vi "main.vi"() -> ()   [LabVIEW 2016, in "LabVIEWCodeCoverage.lvlib"]
uses:
  LabVIEWCodeCoverage.lvlib
panel:
  in  "Reset":bool
  in  "Refresh%":bool
  in  "SourcePath":path
  in  "Stop":bool
  in  "Start":bool
  in  "RefreshContext":bool
  in  "Context":u16(ring) items=["<Empty>", "Main Application Instance", "NI.LV.Merge", "src.lvproj My Computer", "src.lvproj My Computer"]
  in  "VITree":string(tree)
  in  "UnCoveredDiagram":i32(listbox)
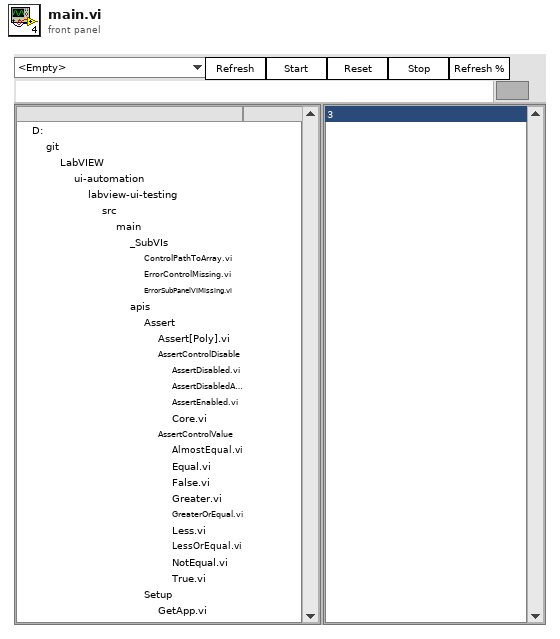
[diagram p1: front panel]
types:
  T1 = enum32{"Invalid", "Standard", "Closed", "Hidden", "Minimized", "Maximized"}
  T2 = enum32{"invalid app kind", "Development System", "Run Time System", "Student Edition", "Embedded LabVIEW", "Evaluation", "Custom"}
  T3 = cluster{"Context":string, "Project":string, "Display":string, "ProjectPath":path}
  T4 = cluster{"Context":string, "Project":string, "Display":string, "ProjectPath":path}[]
  T5 = cluster{"Core":cluster{"Current VI Reference":refnum<vi>, "Close Panel on Exit?":bool}, "ActiveContext":string, "Context[]":cluster{"Context":string, "Project":string, "Display":string, "ProjectPath":path}[], "SourcePath":path, "SourceFiles[]":path[], "ActiveVI":string, "Uncovered Diagrams":refnum<vi>[], "ActiveVIRef":refnum<vi>}
  T6 = cluster{"Current VI Reference":refnum<vi>, "Close Panel on Exit?":bool}
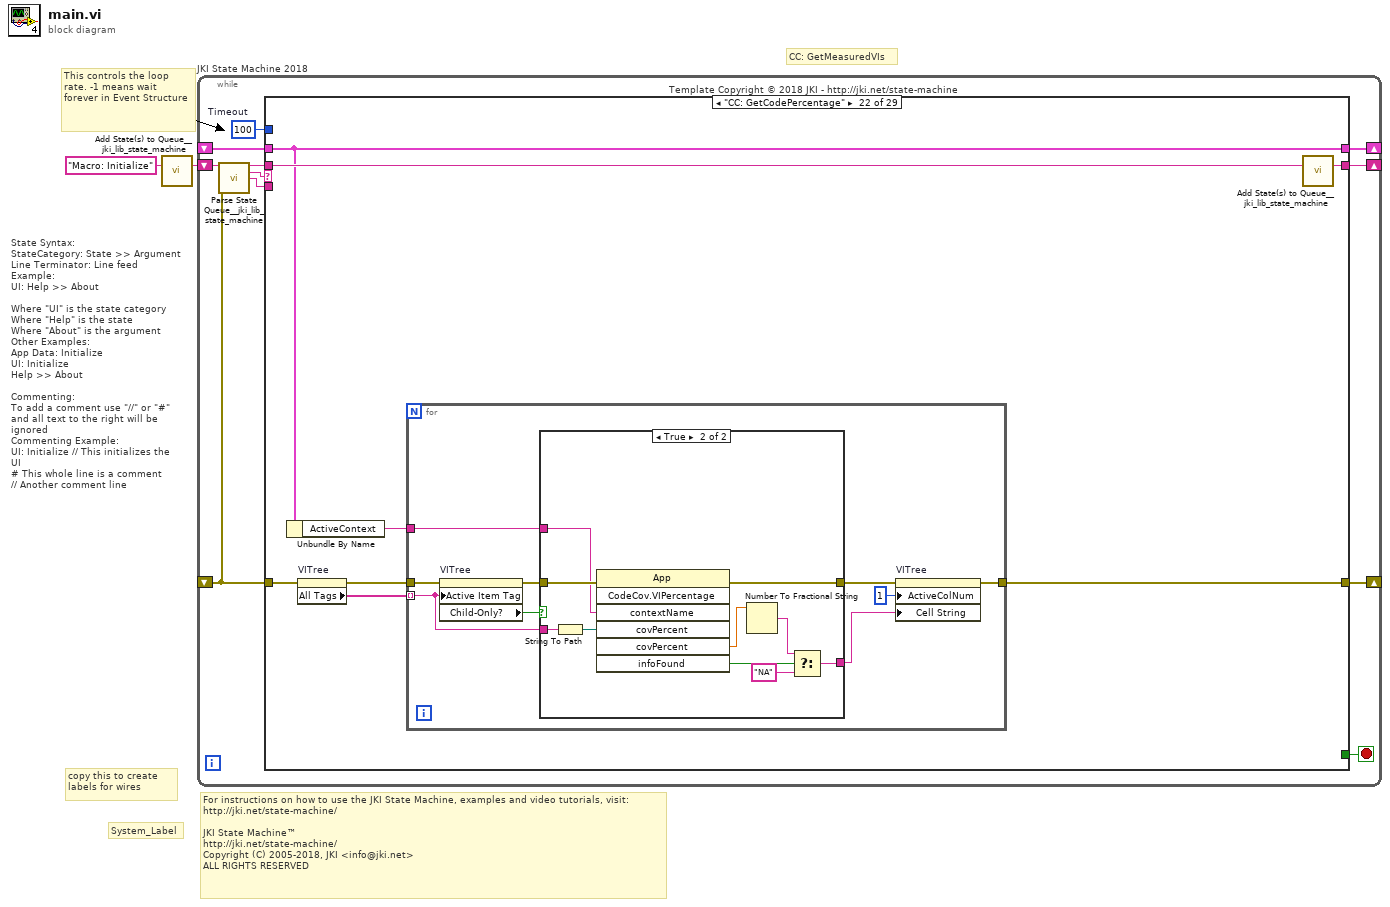
[diagram p0: block diagram]
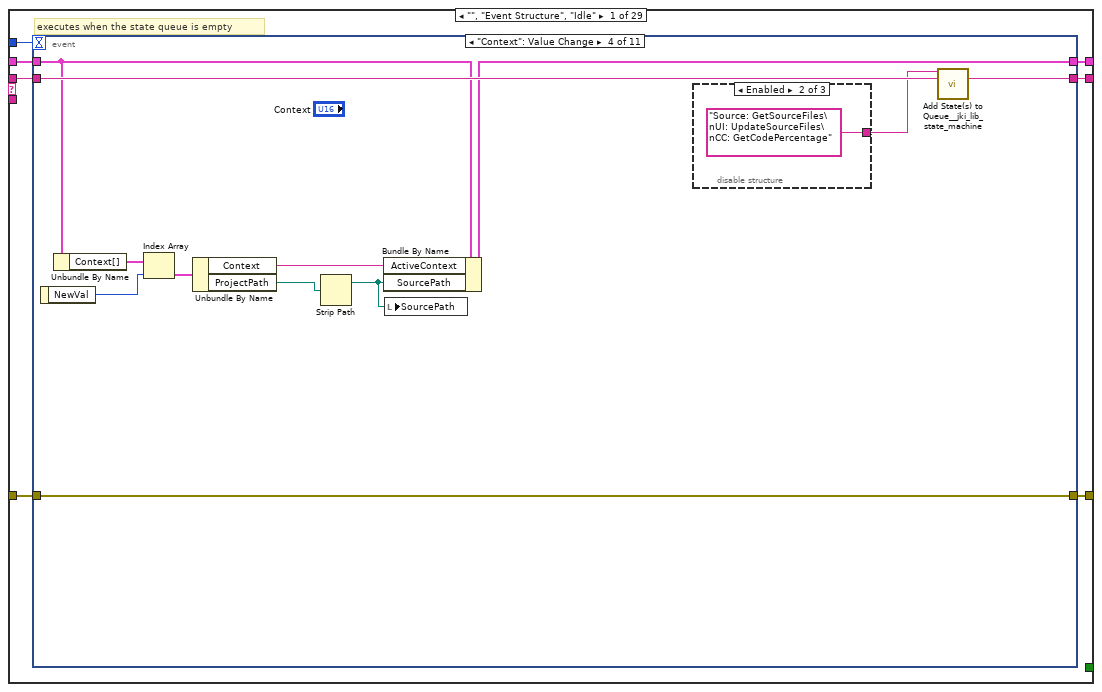
[diagram p2: hidden frame]
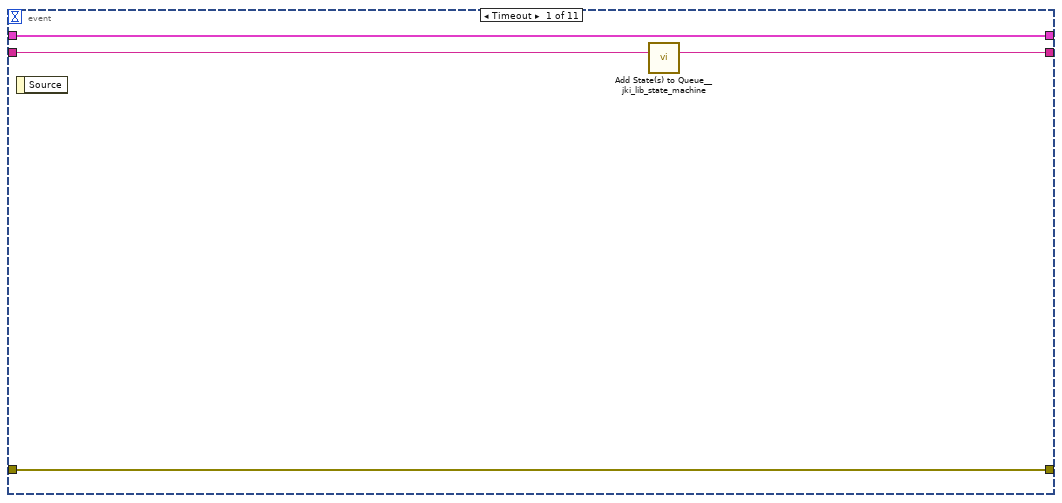
[diagram p3: hidden frame]
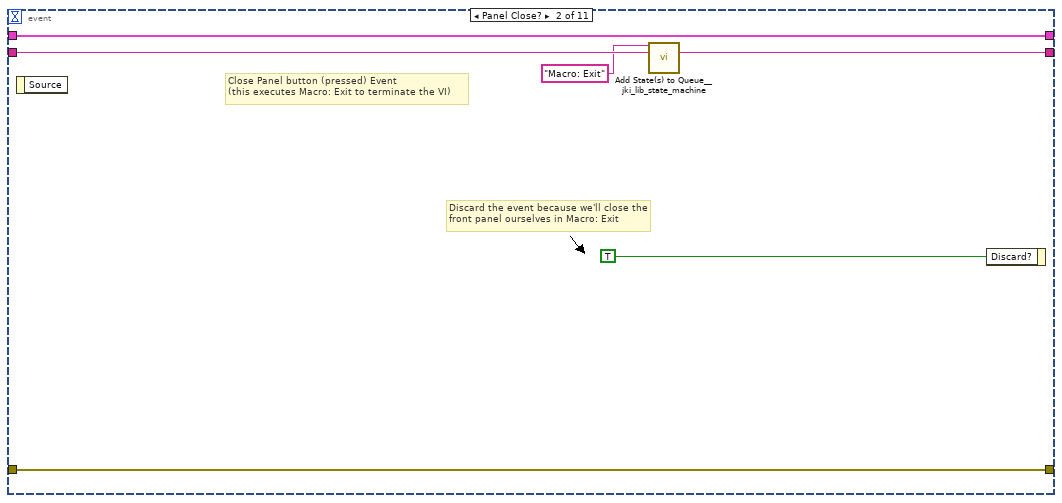
[diagram p4: hidden frame]
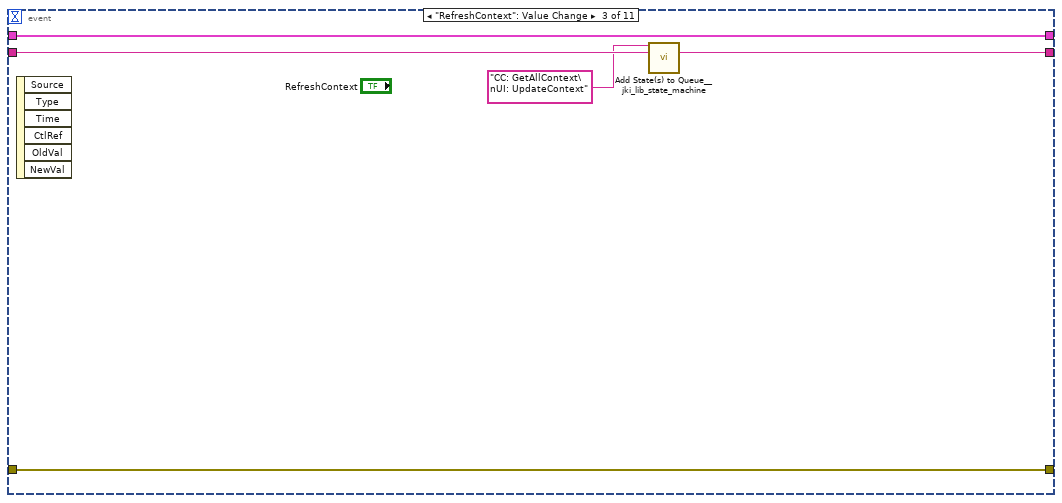
[diagram p5: hidden frame]
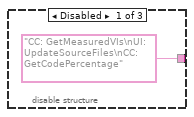
[diagram p6: hidden frame]
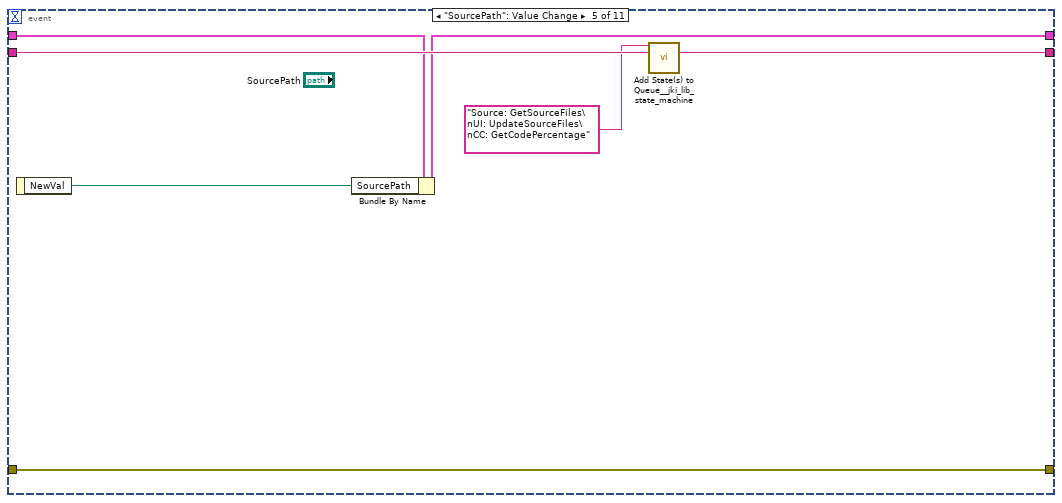
[diagram p8: hidden frame]
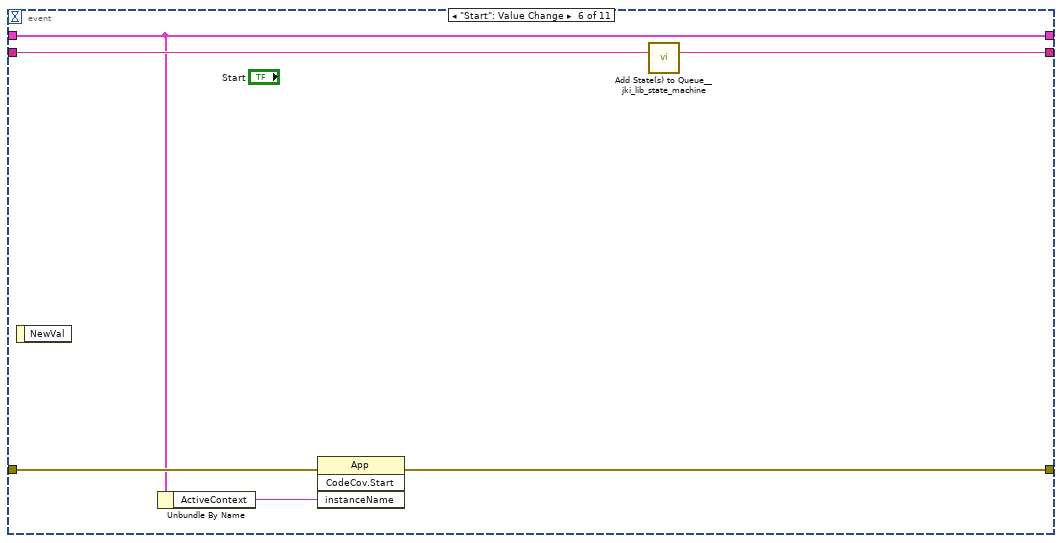
[diagram p9: hidden frame]
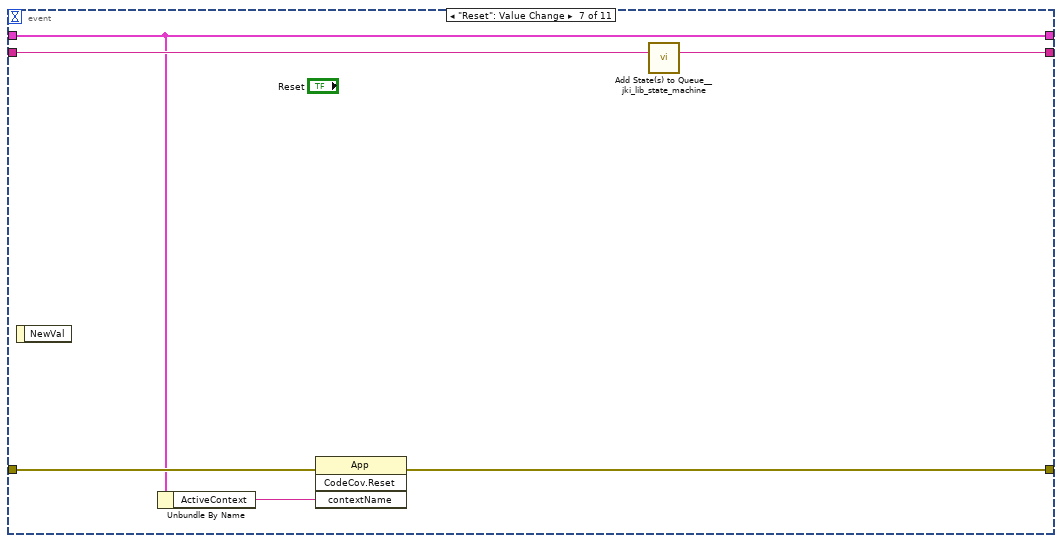
[diagram p10: hidden frame]
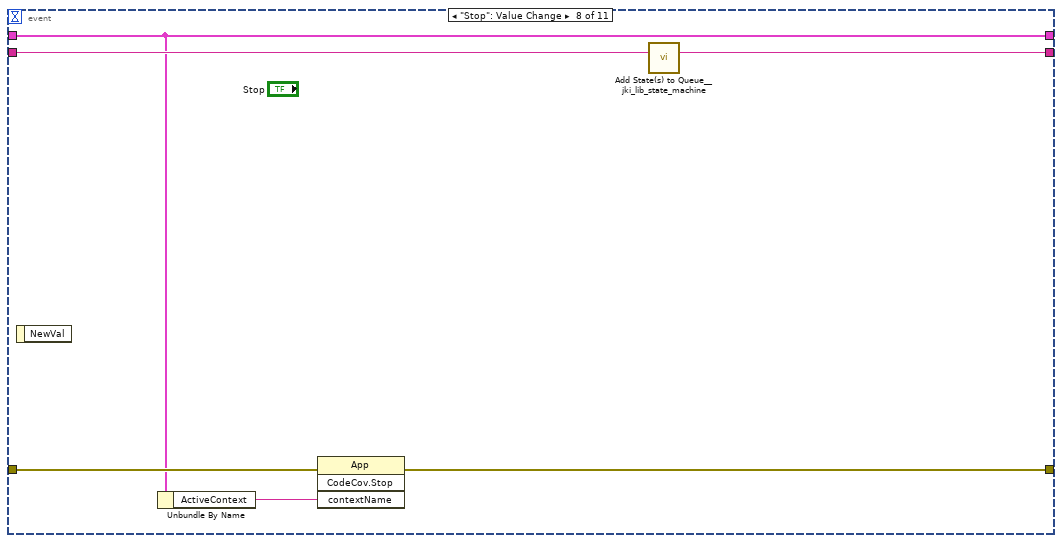
[diagram p11: hidden frame]
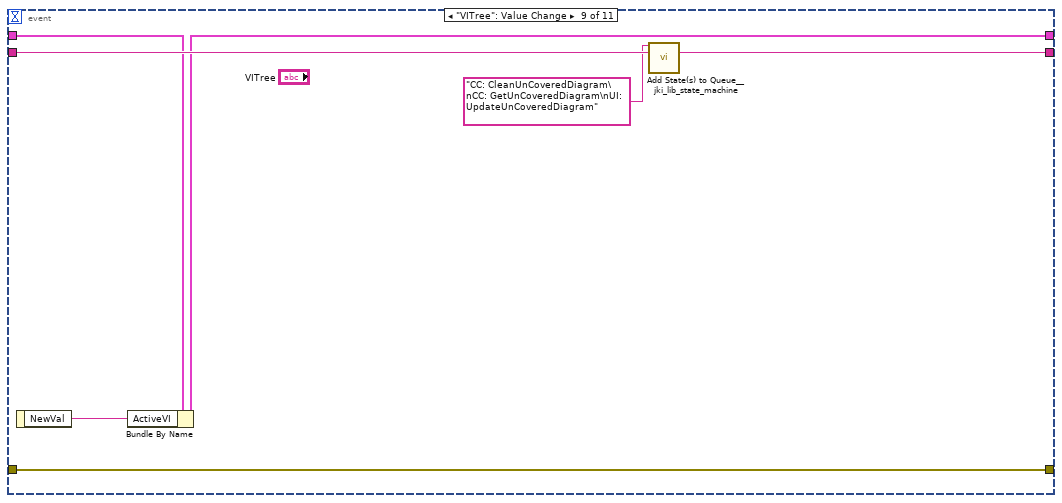
[diagram p12: hidden frame]
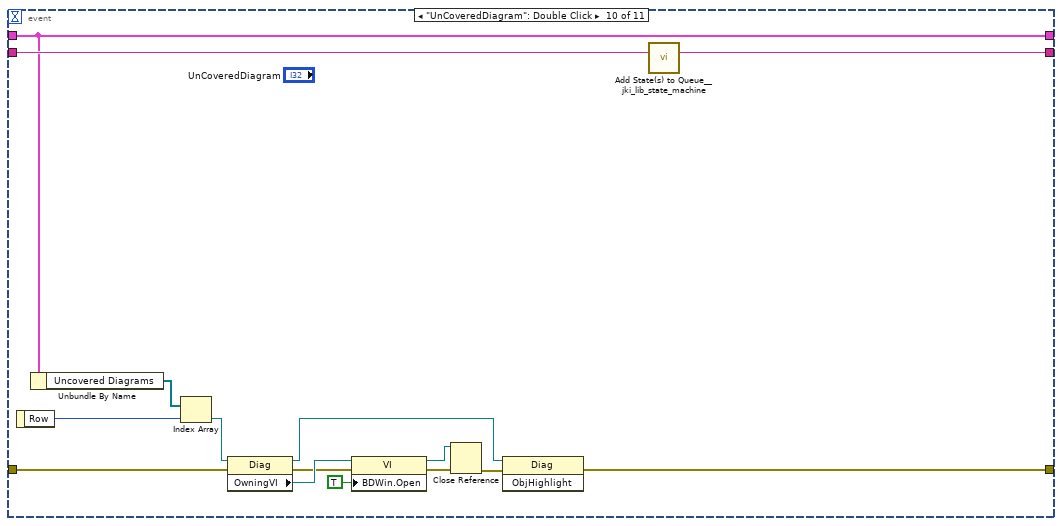
[diagram p13: hidden frame]
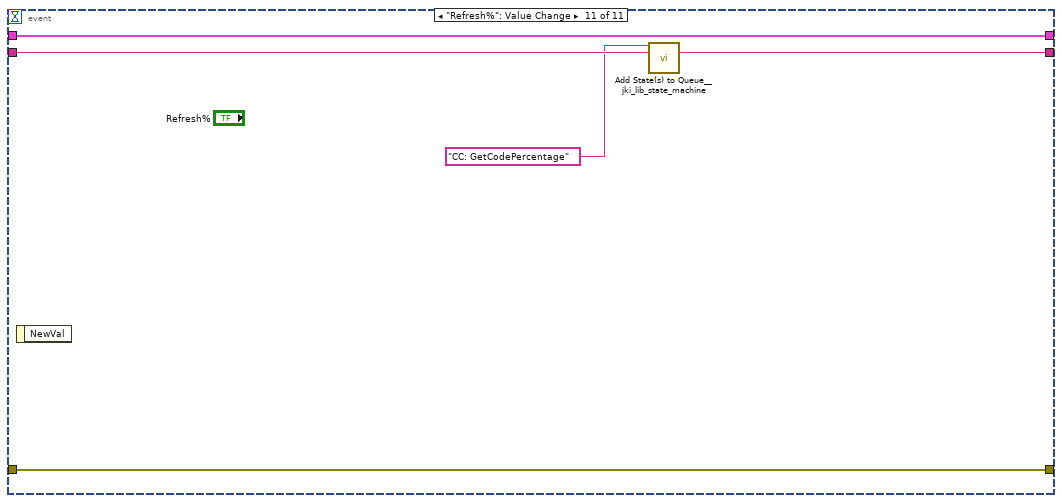
[diagram p14: hidden frame]
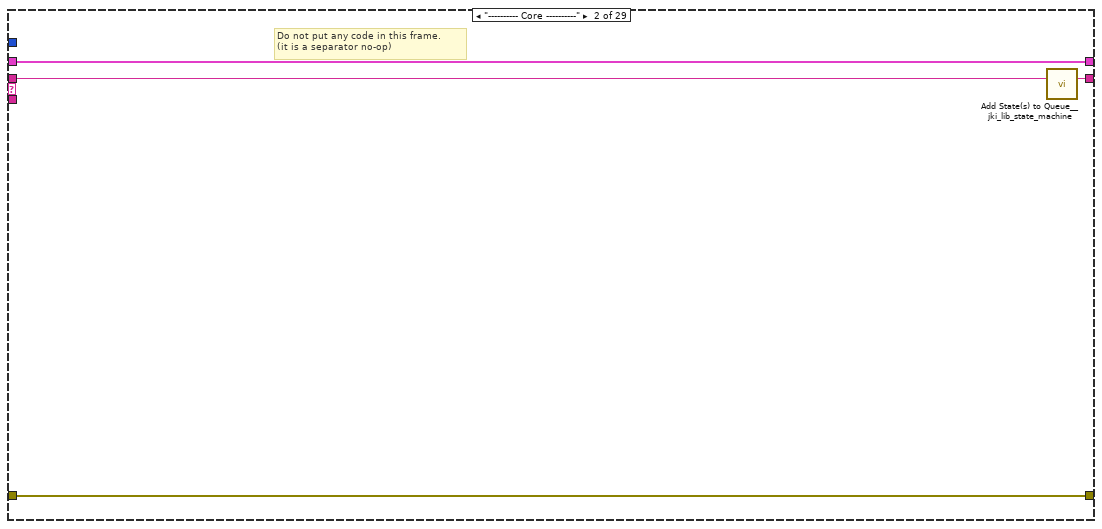
[diagram p15: hidden frame]
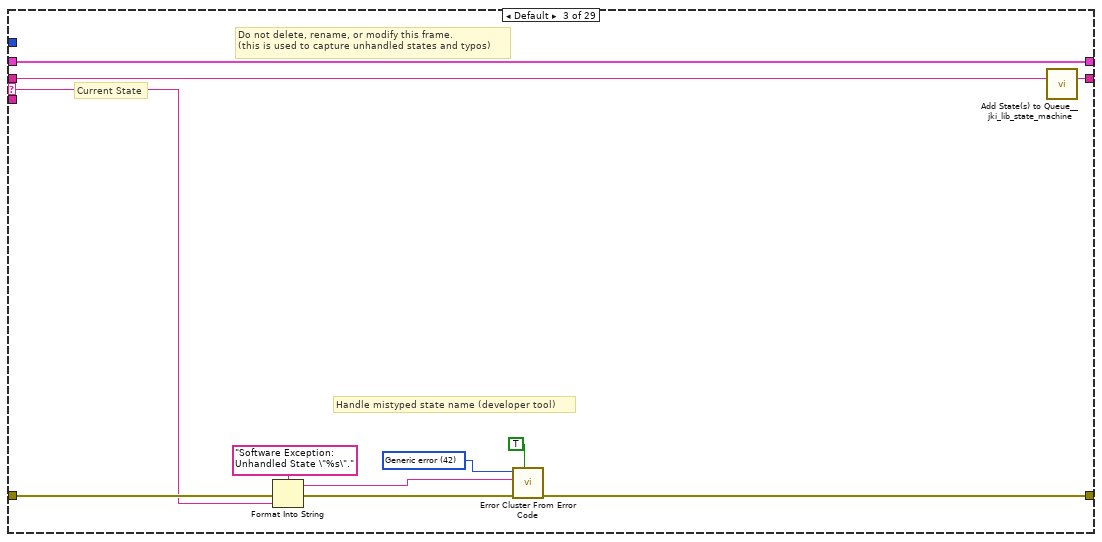
[diagram p16: hidden frame]
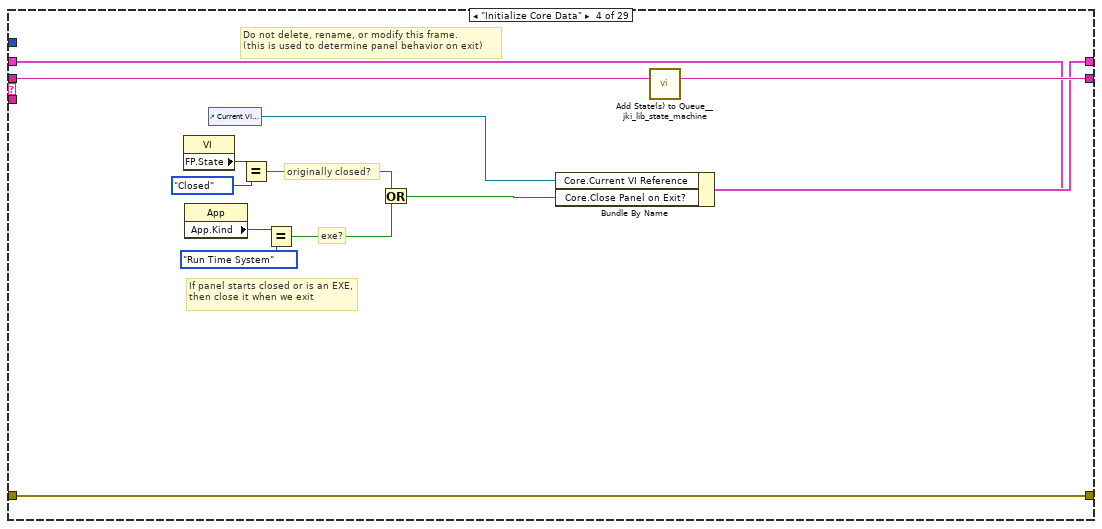
[diagram p17: hidden frame]
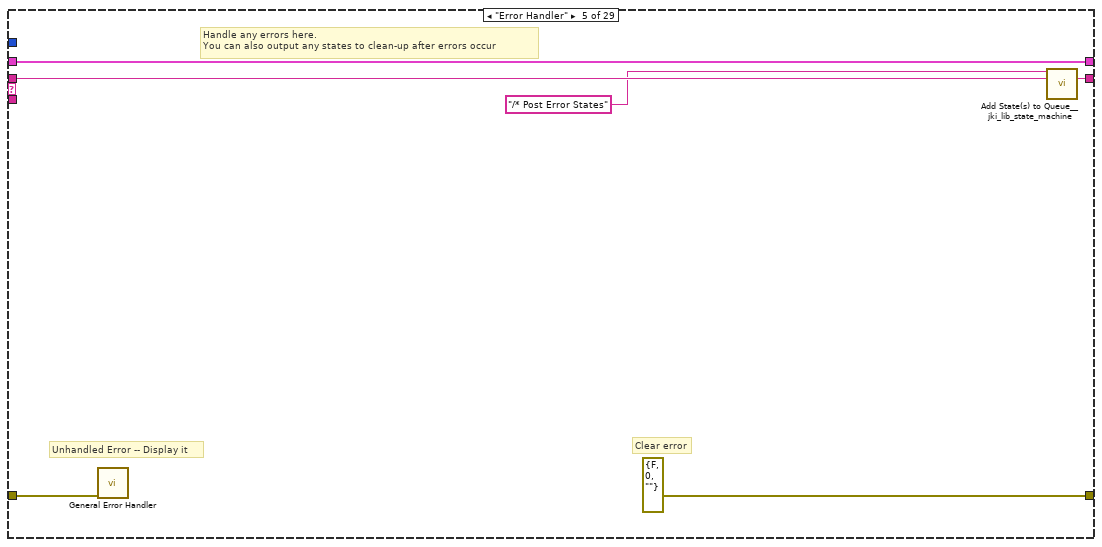
[diagram p18: hidden frame]
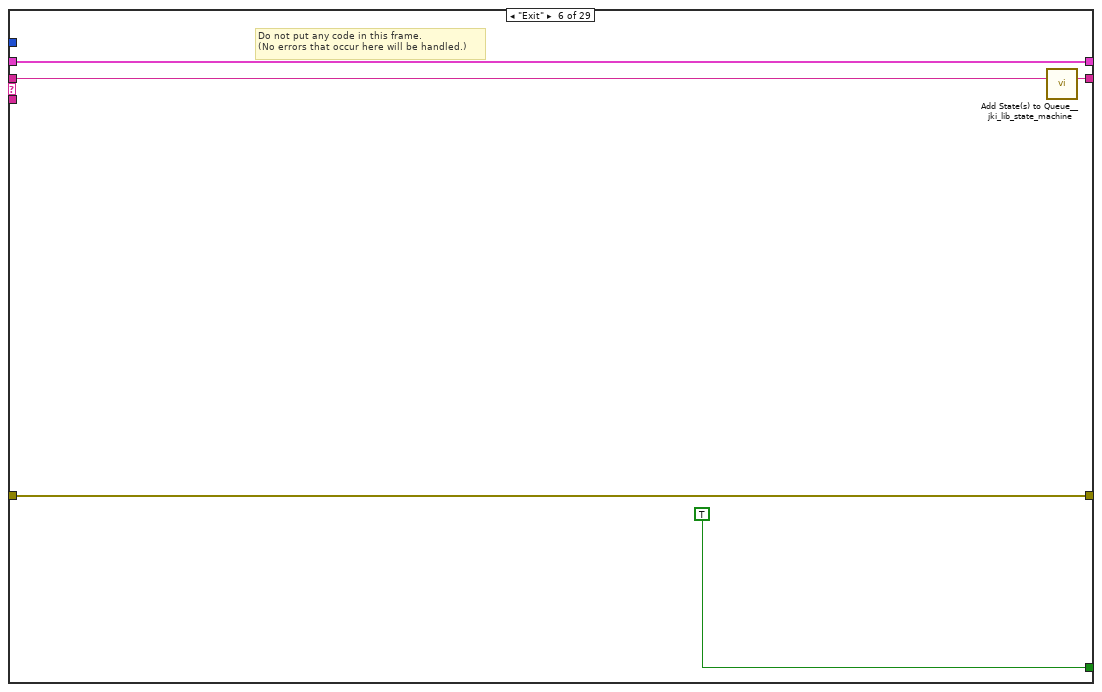
[diagram p19: hidden frame]
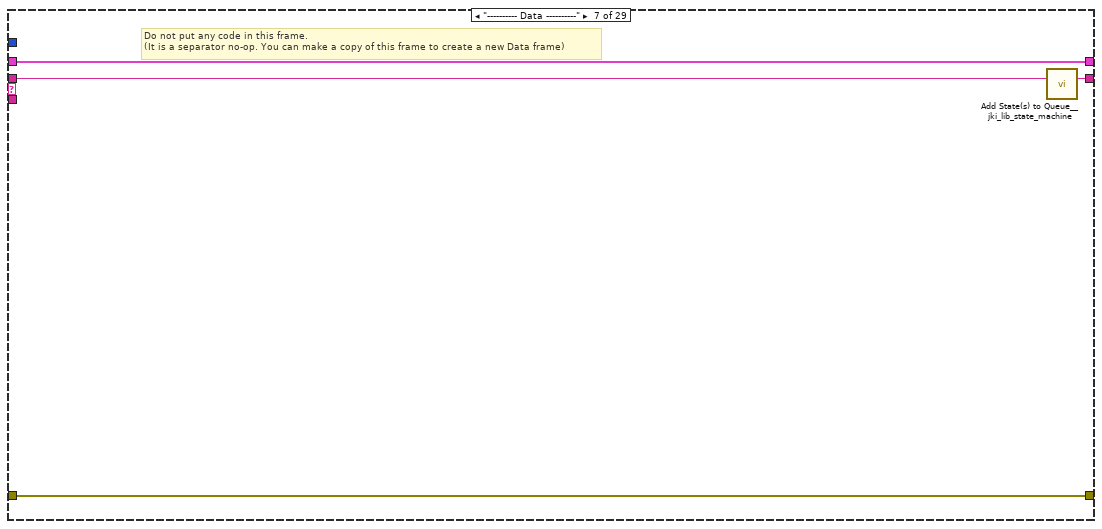
[diagram p20: hidden frame]
diagram:
  # "CC: GetMeasuredVIs"
  # "For instructions on how to use the JKI State Machine, examples and video tutorials, visit:\nhttp://jki.net/state-machine/\n\nJKI State Machine™\nhttp://jki.net/state-machine/\nCopyright (C) 2005-2018, JKI <info@jki.net>\nALL RIGHTS RESERVED"
  # "State Syntax:\nStateCategory: State >> Argument\nLine Terminator: Line feed\nExample:\nUI: Help >> About\n\nWhere \"UI\" is the state category\nWhere \"Help\" is the state\nWhere \"About\" is the argument\nOther Examples:\nApp Data: Initialize\nUI: Initialize\nHelp >> About\n\nCommenting:\nTo add a comment use \"//\" or \"#\" and all text to the right will be ignored\nCommenting Example:\nUI: Initialize // This initializes the UI\n# This whole line is a comment\n// Another comment line"
  # "copy this to create labels for wires"
  # "This controls the loop rate. -1 means wait forever in Event Structure"
  # "System_Label"
  n1 = call <vilib>:"Add State(s) to Queue__jki_lib_state_machine.vi"("State(s) in (\"\")"="Macro: Initialize") -> ("States Out"=w2:string)  [unwired: 14 in]
  n2 = while "JKI State Machine 2018" {
    shift-right: [w6] -> _
    shift-left: _ -> [w5]
    shift-right: [w9] -> _
    shift-left: _ -> [w3]
    shift-right: [w8] -> _
    shift-left: w2 -> [w10]
    stop <- w7 stop-if-true
    w4 = 100  # Timeout
    # "Template Copyright © 2018 JKI - http://jki.net/state-machine"
    n3 = call <vilib>:"Parse State Queue__jki_lib_state_machine.vi"("State Queue"=w10, "Error In (no error)"=w3) -> ("Remaining States"=w12:string, "Current State"=w13:string, "Arguments"=w11:string)  [unwired: 11 in]
    n4 = case shown="\"CC: GetCodePercentage\"" w13 {
      selector: w13 -> [_ _ w106 _ _ _ _ _ _ _ _ _ _ _ _ _ _ _ _ _ _ _ _ _ _ _ _ _ _]
      tunnel: w12 -> [w20 w105 w110 w129 w135 w140 w144 w156 w162 w166 w173 w179 w190 w262 w283 w302 w312 w317 w327 w331 w346 w362 w392 w421 w425 w429 w433 w444 w459]
      tunnel: w11 -> [_ _ _ _ _ _ _ _ _ _ _ w174 w184 _ _ _ _ _ _ _ _ _ _ _ _ _ _ _ _]
      tunnel: w5 -> [w18 w102 w108 w122 w132 w138 w141 _ w157 w163 w170 w177 w186 w260 w281 w300 w309 w314 w324 w328 w343 w356 w389 w419 w422 w426 w430 w442 w454]
      tunnel: [w17 w103 w112 w126 errorcluster {"status"=FALSE, "code"=0, "source"=""} ("error out") w137 w142 w153 w158 w164 w171 w175 w187 w258 w267 w299 w310 w315 w325 w329 w340 w360 w388 w410 w423 w427 w431 w436 w455] -> w9
      tunnel: w3 -> [w16 w103 w111 w126 w131 w137 w142 w153 w159 w164 w171 w176 w188 w259 w279 w298 w310 w315 w325 w329 w344 w359 w390 w417 w423 w427 w431 w441 w456]
      tunnel: [w19 w104 w109 w128 w134 w139 w143 w155 w161 w165 w172 w178 w189 w261 w282 w301 w311 w316 w326 w330 w345 w361 w391 w420 w424 w428 w432 w443 w458] -> w8
      tunnel: [_ _ _ _ _ TRUE _ _ _ _ _ _ _ _ _ _ _ _ _ _ _ _ _ _ _ _ _ _ _] -> w7
      tunnel: [w15 w102 w108 w127 w132 w138 w141 w154 w157 w163 w170 w177 w186 w260 w281 w300 w309 w314 w324 w328 w341 w356 w387 w418 w422 w426 w430 w437 w457] -> w6
      tunnel: w4 -> [w14 _ _ _ _ _ _ _ _ _ _ _ _ _ _ _ _ _ _ _ _ _ _ _ _ _ _ _ _]
      frame "", "Event Structure", "Idle" {
        # "executes when the state queue is empty"
        n5 = event shown="[3] \"Context\": Value Change" {
          selector: _ -> [_ _ _ _ _ _ _ _ _ _ _]
          dyn-events: _ -> [_ _ _ _ _ _ _ _ _ _ _]
          timeout: w14 -> [_ _ _ _ _ _ _ _ _ _ _]
          tunnel: w20 -> [w24 w30 w35 w47 w56 w62 w68 w74 w81 w96 w101]
          tunnel: [w23 w29 w34 w46 w55 w61 w67 w73 w80 w95 w100] -> w19
          tunnel: w18 -> [w21 w27 w32 w43 w52 w58 w64 w70 w78 w94 w98]
          tunnel: [w22 w28 w33 w45 w54 w59 w65 w71 w79 w91 w99] -> w17
          tunnel: w16 -> [w22 w28 w33 w45 w54 w60 w66 w72 w79 w90 w99]
          tunnel: [w21 w27 w32 w44 w53 w58 w64 w70 w77 w94 w98] -> w15
          event Timeout {
            n6 = event-data() -> ()  [unwired: 1 in, 1 out]
            n7 = call <vilib>:"Add State(s) to Queue__jki_lib_state_machine.vi"("State(s) in (\"\")"=w24) -> ("States Out"=w23:string)  [unwired: 14 in]
          }
          event Panel Close? {
            # "Discard the event because we'll close the front panel ourselves in Macro: Exit"
            # "Close Panel button (pressed) Event\n(this executes Macro: Exit to terminate the VI)"
            n8 = event-data() -> ()  [unwired: 1 in, 1 out]
            n9 = call <vilib>:"Add State(s) to Queue__jki_lib_state_machine.vi"("State(s) in Front (\"\")"="Macro: Exit", "State(s) in (\"\")"=w30) -> ("States Out"=w29:string)  [unwired: 13 in]
            n10 = event-data("Discard?"=TRUE) -> ()  [unwired: 1 in, 1 out]
          }
          event "RefreshContext": Value Change {
            n11 = event-data() -> ()  [unwired: 1 in, 6 out]
            n12 = call <vilib>:"Add State(s) to Queue__jki_lib_state_machine.vi"("State(s) in Front (\"\")"="CC: GetAllContext\nUI: UpdateContext", "State(s) in (\"\")"=w35) -> ("States Out"=w34:string)  [unwired: 13 in]
          }
          event "Context": Value Change {
            n13 = event-data() -> ("NewVal"=w36:u16)  [unwired: 1 in]
            n14 = Unbundle By Name(w43) -> ("Context[]"=w37:T4)
            n15 = Index Array(array=w37, index=w36) -> (element=w42:T3)
            n16 = Unbundle By Name(w42) -> ("Context"=w41:string, "ProjectPath"=w39:path)
            n17 = Strip Path(path=w39) -> (stripped path=w38:path)  [unwired: 1 out]
            n18 = Bundle By Name(cluster=w43, "ActiveContext"=w41, "SourcePath"=w38) -> (w44:T5)
            n19 = local write "SourcePath"(w38) -> ()
            n20 = disable-structure shown="Enabled" {
              disable-tunnel: ["CC: GetMeasuredVIs\nUI: UpdateSourceFiles\nCC: GetCodePercentage" "Source: GetSourceFiles\nUI: UpdateSourceFiles\nCC: GetCodePercentage" _] -> w40
              frame Disabled {
              }
              frame Enabled {
              }
              frame Disabled {
              }
            }
            n21 = call <vilib>:"Add State(s) to Queue__jki_lib_state_machine.vi"("State(s) in Front (\"\")"=w40, "State(s) in (\"\")"=w47) -> ("States Out"=w46:string)  [unwired: 13 in]
          }
          event "SourcePath": Value Change {
            n22 = event-data() -> ("NewVal"=w51:path)  [unwired: 1 in]
            n23 = Bundle By Name(cluster=w52, "SourcePath"=w51) -> (w53:T5)
            n24 = call <vilib>:"Add State(s) to Queue__jki_lib_state_machine.vi"("State(s) in Front (\"\")"="Source: GetSourceFiles\nUI: UpdateSourceFiles\nCC: GetCodePercentage", "State(s) in (\"\")"=w56) -> ("States Out"=w55:string)  [unwired: 13 in]
          }
          event "Start": Value Change {
            n25 = event-data() -> ()  [unwired: 1 in, 1 out]
            n26 = Unbundle By Name(w58) -> ("ActiveContext"=w57:string)
            n27 = invoke class="App" method="CodeCov.Start"(error in=w60, "instanceName"=w57) -> (error out=w59:errorcluster)  [unwired: 2 in, 3 out]
            n28 = call <vilib>:"Add State(s) to Queue__jki_lib_state_machine.vi"("State(s) in (\"\")"=w62) -> ("States Out"=w61:string)  [unwired: 14 in]
          }
          event "Reset": Value Change {
            n29 = event-data() -> ()  [unwired: 1 in, 1 out]
            n30 = Unbundle By Name(w64) -> ("ActiveContext"=w63:string)
            n31 = invoke class="App" method="CodeCov.Reset"(error in=w66, "contextName"=w63) -> (error out=w65:errorcluster)  [unwired: 2 in, 3 out]
            n32 = call <vilib>:"Add State(s) to Queue__jki_lib_state_machine.vi"("State(s) in (\"\")"=w68) -> ("States Out"=w67:string)  [unwired: 14 in]
          }
          event "Stop": Value Change {
            n33 = event-data() -> ()  [unwired: 1 in, 1 out]
            n34 = Unbundle By Name(w70) -> ("ActiveContext"=w69:string)
            n35 = invoke class="App" method="CodeCov.Stop"(error in=w72, "contextName"=w69) -> (error out=w71:errorcluster)  [unwired: 2 in, 3 out]
            n36 = call <vilib>:"Add State(s) to Queue__jki_lib_state_machine.vi"("State(s) in (\"\")"=w74) -> ("States Out"=w73:string)  [unwired: 14 in]
          }
          event "VITree": Value Change {
            n37 = event-data() -> ("NewVal"=w76:string)  [unwired: 1 in]
            n38 = Bundle By Name(cluster=w78, "ActiveVI"=w76) -> (w77:T5)
            n39 = call <vilib>:"Add State(s) to Queue__jki_lib_state_machine.vi"("State(s) in Front (\"\")"="CC: CleanUnCoveredDiagram\nCC: GetUnCoveredDiagram\nUI: UpdateUnCoveredDiagram", "State(s) in (\"\")"=w81) -> ("States Out"=w80:string)  [unwired: 13 in]
          }
          event "UnCoveredDiagram": Double Click {
            n40 = event-data() -> ("Row"=w92:i32)  [unwired: 1 in]
            n41 = Unbundle By Name(w94) -> ("Uncovered Diagrams"=w93:refnum<vi>[])
            n42 = Index Array(array=w93, index=w92) -> (element=w83:refnum<vi>)
            n43 = property class="Diag"(reference=w83, error in=w90) -> (reference out=w82:refnum<vi>, error out=w88:errorcluster, "OwningVI"=w89:refnum<vi>)
            n44 = property class="VI"(reference=w89, error in=w88, "BDWin.Open"=TRUE ("Block Diagram Window:Open")) -> (reference out=w85:refnum<vi>, error out=w86:errorcluster)
            n45 = Close Reference(reference=w85, error in (no error)=w86) -> (error out=w84:errorcluster)
            n46 = invoke class="Diag" method="ObjHighlight"(reference=w82, error in=w84) -> (error out=w91:errorcluster)  [unwired: 1 in, 2 out]
            n47 = call <vilib>:"Add State(s) to Queue__jki_lib_state_machine.vi"("State(s) in (\"\")"=w96) -> ("States Out"=w95:string)  [unwired: 14 in]
          }
          event "Refresh%": Value Change {
            n48 = event-data() -> ()  [unwired: 1 in, 1 out]
            n49 = call <vilib>:"Add State(s) to Queue__jki_lib_state_machine.vi"("State(s) in Front (\"\")"="CC: GetCodePercentage", "State(s) in (\"\")"=w101) -> ("States Out"=w100:string)  [unwired: 13 in]
          }
        }
      }
      frame "---------- Core ----------" {
        # "Do not put any code in this frame.\n(it is a separator no-op)"
        n50 = call <vilib>:"Add State(s) to Queue__jki_lib_state_machine.vi"("State(s) in (\"\")"=w105) -> ("States Out"=w104:string)  [unwired: 14 in]
      }
      frame Default {
        w115 = 42 items=["No error", "Argument error", "Memory is full", "Out of zone", "End of file", "File already open", "Generic file I/O error", "File not found", "File permission error", "Disk is full", "Duplicate path", "Too many files open", "System feature not enabled", "Resource file not found", "Cannot add resource", "Resource not found", "Image not found", "Image memory error", "Pen does not exist", "Config type invalid", "Config token not found", "Config parse error", "Config memory error", "Bad external code format", "Bad external code offset", "External code not present", "Null window", "Destroy window error", "Null menu", "Print aborted", "Bad print record", "Print driver error", "Windows error during printing", "Memory error during printing", "Print dialog error", "Generic print error", "Invalid device refnum", "Device not found", "Device parameter error", "Device unit error", "Cannot open device", "Device call aborted", "Generic error", "Cancelled by user", "Object ID too low", "Object ID too high", "Object not in heap", "Unknown heap", "Unknown object (invalid DefProc)", "Unknown object (DefProc not in table)", "Message out of range", "Invalid (null) method", "Unknown message", "Manager call not supported", "Bad address", "Network operation in progress", "Network operation timed out", "Connection is busy", "Network attribute not supported", "Network error", "Address in use", "System out of memory", "Connection aborted", "Connection refused", "Not connected", "Already connected", "Connection closed", "Initialization error (interapplication manager)", "Bad occurrence", "Wait on unbound occurrence handler", "Occurrence queue overflow", "Datalog type conflict", "Unused", "Unrecognized type (interapplication manager)", "Memory corrupt", "Failed to make temporary DLL", "Old CIN version", "Drag socket not found", "Failed to load drop-object", "Failed to register OLE object", "Failed to release OLE object", "Format specifier type mismatch", "Unknown format specifier", "Too few format specifiers", "Too many format specifiers", "Scan failed", "Newer CIN version", "Error converting to variant", "Runtime menu error", "Password tampered", "Variant attribute not found", "Incompatible variant data type", "Event data is not available", "Event Store is not present", "Occurrence is not found", "Event Queue is not created", "Event info is not available", "Refnum passed is NULL", "Error retrieving Class GUID", "Error retrieving CoClass GUID", "Error retrieving TypeLib GUID.", "Bad built application magic bytes.", "Specific driver is different from the specific driver associated with the Logical Name.", "There is no session opened to the class driver.", "Max Error", "MAX - Error with config objects", "MAX - Error loading configuration", "MAX - Group not supported"]
        # "Current State"
        # "Do not delete, rename, or modify this frame.\n(this is used to capture unhandled states and typos)"
        # "Handle mistyped state name (developer tool)"
        n51 = Format Into String(format string="Software Exception: Unhandled State \"%s\"." ("message"), error in=w111, w106) -> (resulting string=w114:string, error out=w113:errorcluster)  [unwired: 1 in]
        n52 = call <vilib>:"Error Cluster From Error Code.vi"("show call chain? (False)"=TRUE, "error in (no error)"=w113, "error message (\"\")"=w114, "error code (0)"=w115) -> ("error out"=w112:errorcluster)  [unwired: 5 in]
        n53 = call <vilib>:"Add State(s) to Queue__jki_lib_state_machine.vi"("State(s) in (\"\")"=w110) -> ("States Out"=w109:string)  [unwired: 14 in]
      }
      frame "Initialize Core Data" {
        # "Do not delete, rename, or modify this frame.\n(this is used to determine panel behavior on exit)"
        # "originally closed?"
        # "exe?"
        # "If panel starts closed or is an EXE, then close it when we exit"
        n54 = property class="VI"() -> ("FP.State"=w119:T1)  [unwired: 2 in, 2 out]
        n55 = property class="App"() -> ("App.Kind"=w125:T2)  [unwired: 2 in, 2 out]
        n56 = control-ref of="Current VI Reference"() -> (w120:refnum<vi>)
        n57 = Equal?(x=w119, y=T1."Closed" ("Front Panel Window:State")) -> (x = y?=w117:bool)
        n58 = Equal?(x=w125, y=T2."Run Time System" ("Application:Kind")) -> (x = y?=w123:bool)
        n59 = Or(x=w117, y=w123) -> (x .or. y?=w121:bool)
        n60 = Bundle By Name(cluster=w122, "Core.Current VI Reference"=w120, "Core.Close Panel on Exit?"=w121) -> (w127:T5)
        n61 = call <vilib>:"Add State(s) to Queue__jki_lib_state_machine.vi"("State(s) in (\"\")"=w129) -> ("States Out"=w128:string)  [unwired: 14 in]
      }
      frame "Error Handler" {
        # "Unhandled Error -- Display it"
        # "Handle any errors here.\nYou can also output any states to clean-up after errors occur"
        # "Clear error"
        n62 = call <vilib>:"General Error Handler.vi"("error in (no error)"=w131) -> ()  [unwired: 10 in, 5 out]
        n63 = call <vilib>:"Add State(s) to Queue__jki_lib_state_machine.vi"("State(s) in Front (\"\")"="/* Post Error States", "State(s) in (\"\")"=w135) -> ("States Out"=w134:string)  [unwired: 13 in]
      }
      frame "Exit" {
        # "Do not put any code in this frame.\n(No errors that occur here will be handled.)"
        n64 = call <vilib>:"Add State(s) to Queue__jki_lib_state_machine.vi"("State(s) in (\"\")"=w140) -> ("States Out"=w139:string)  [unwired: 14 in]
      }
      frame "---------- Data ----------" {
        # "Do not put any code in this frame.\n(It is a separator no-op. You can make a copy of this frame to create a new Data frame)"
        n65 = call <vilib>:"Add State(s) to Queue__jki_lib_state_machine.vi"("State(s) in (\"\")"=w144) -> ("States Out"=w143:string)  [unwired: 14 in]
      }
      frame "Data: Initialize" {
        w145 = refnum<vi> refnum  # ActiveVIRef
        w146 = refnum<vi>[] []  # Uncovered Diagrams
        w147 = ""  # ActiveVI
        w149 = path[] []  # SourceFiles[]
        w148 = path ""  # SourcePath
        w150 = T4 []  # Context[]
        w151 = ""  # ActiveContext
        w152 = T6 {"Current VI Reference"=refnum, "Close Panel on Exit?"=FALSE}  # Core
        # "do not delete - used by framework"
        # "Data names and types of shift register data are defined by this bundle."
        # "Initialize the shift-register data, here.\n(data names are defined by what you wire into the bundle function)"
        n66 = Bundle("Core"=w152, "ActiveContext"=w151, "Context[]"=w150, "SourcePath"=w148, "SourceFiles[]"=w149, "ActiveVI"=w147, "Uncovered Diagrams"=w146, "ActiveVIRef"=w145) -> (w154:T5)  [unwired: 1 in]
        n67 = call <vilib>:"Add State(s) to Queue__jki_lib_state_machine.vi"("State(s) in (\"\")"=w156) -> ("States Out"=w155:string)  [unwired: 14 in]
      }
      frame "Data: Cleanup" {
        # "Cleanup any data and references, here.\n(this is called automatically, by the Macro: Exit)"
        n68 = Unbundle By Name(w157) -> ("Core.Current VI Reference"=w160:refnum<vi>)
        n69 = Close Reference(reference=w160, error in (no error)=w159) -> (error out=w158:errorcluster)
        n70 = call <vilib>:"Add State(s) to Queue__jki_lib_state_machine.vi"("State(s) in (\"\")"=w162) -> ("States Out"=w161:string)  [unwired: 14 in]
      }
      frame "---------- UI ----------" {
        # "Do not put any code in this frame.\n(It is a separator no-op. You can make a copy of this frame to create a new UI frame)"
        n71 = call <vilib>:"Add State(s) to Queue__jki_lib_state_machine.vi"("State(s) in (\"\")"=w166) -> ("States Out"=w165:string)  [unwired: 14 in]
      }
      frame "UI: Initialize" {
        # "Initialize the User Interface, here.\n(this is called automatically, by the Macro: Init)"
        n72 = Unbundle By Name(w170) -> ("SourcePath"=w169:path, "ActiveVI"=w168:string)
        n73 = local write "SourcePath"(w169) -> ()
        n74 = local write "VITree"(w168) -> ()
        n75 = local write "Context"(0) -> ()
        n76 = call <vilib>:"Add State(s) to Queue__jki_lib_state_machine.vi"("State(s) in (\"\")"=w173) -> ("States Out"=w172:string)  [unwired: 14 in]
      }
      frame "UI: Cursor Set" {
        # "Argument"
        # "Set and Unset Cursor Busy.\n(Usage: \"UI: Cursor Set >> Busy|Idle\")"
        n77 = case shown="\"Idle\", Default" w174 {
          tunnel: w176 -> [w181 w183]
          tunnel: [w180 w182] -> w175
          frame "Idle", Default {
            n78 = call <vilib>:"Unset Busy.vi"("error in (no error)"=w181) -> ("error out"=w180:errorcluster)  [unwired: 10 in]
          }
          frame "Busy" {
            n79 = call <vilib>:"Set Busy.vi"("error in (no error)"=w183) -> ("error out"=w182:errorcluster)  [unwired: 9 in, 1 out]
          }
        }
        n80 = call <vilib>:"Add State(s) to Queue__jki_lib_state_machine.vi"("State(s) in (\"\")"=w179) -> ("States Out"=w178:string)  [unwired: 14 in]
      }
      frame "UI: Front Panel State" {
        # "Argument"
        # "Set Front Panel Open or Closed\n(Usage: \"UI: Front Panel State >> Open|Close\")"
        n81 = Unbundle By Name(w186) -> ("Core.Current VI Reference"=w185:refnum<vi>)
        n82 = case shown="\"Hidden\", \"Hide\"" w184 {
          tunnel: w188 -> [w196 w211 w222 w235 w248]
          tunnel: [w198 w212 w224 w237 w250] -> w187
          tunnel: w185 -> [w197 w209 w223 w236 w249]
          frame "Open", "Standard", Default {
            w191 = T1."Standard" ("State")
            n83 = property class="VI"(reference=w197, error in=w196) -> (reference out=w194:refnum<vi>, error out=w195:errorcluster, "FP.State"=w193:T1)
            n84 = Not Equal?(x=w193, y=w191) -> (x != y?=w192:bool)
            n85 = case shown="True" w192 {
              tunnel: [w202 w204] -> w198
              tunnel: w195 -> [w201 w204]
              tunnel: w194 -> [w200 _]
              tunnel: w191 -> [w199 _]
              frame True {
                n86 = invoke class="VI" method="FP.Open"(reference=w200, error in=w201, "Activate"=TRUE, "State"=w199) -> (error out=w202:errorcluster)  [unwired: 1 in, 4 out]
              }
              frame False {
              }
            }
          }
          frame "Close", "Closed" {
            n87 = property class="VI"(reference=w209, error in=w211) -> (reference out=w208:refnum<vi>, error out=w210:errorcluster, "FP.State"=w206:T1)
            n88 = Not Equal?(x=w206, y=T1."Closed" ("Front Panel Window:State")) -> (x != y?=w205:bool)
            n89 = case shown="True" w205 {
              tunnel: [w213 w216] -> w212
              tunnel: w210 -> [w213 w215]
              tunnel: w208 -> [_ w214]
              frame False {
              }
              frame True {
                n90 = invoke class="VI" method="FP.Close"(reference=w214, error in=w215) -> (error out=w216:errorcluster)  [unwired: 1 in, 2 out]
              }
            }
          }
          frame "Hidden", "Hide" {
            w217 = T1."Hidden" ("State")
            n91 = property class="VI"(reference=w223, error in=w222) -> (reference out=w220:refnum<vi>, error out=w221:errorcluster, "FP.State"=w219:T1)
            n92 = Not Equal?(x=w219, y=w217) -> (x != y?=w218:bool)
            n93 = case shown="True" w218 {
              tunnel: [w228 w229] -> w224
              tunnel: w221 -> [w227 w229]
              tunnel: w220 -> [w226 _]
              tunnel: w217 -> [w225 _]
              frame True {
                n94 = invoke class="VI" method="FP.Open"(reference=w226, error in=w227, "State"=w225) -> (error out=w228:errorcluster)  [unwired: 2 in, 4 out]
              }
              frame False {
              }
            }
          }
          frame "Minimize", "Minimized" {
            w230 = T1."Minimized" ("State")
            n95 = property class="VI"(reference=w236, error in=w235) -> (reference out=w233:refnum<vi>, error out=w234:errorcluster, "FP.State"=w232:T1)
            n96 = Not Equal?(x=w232, y=w230) -> (x != y?=w231:bool)
            n97 = case shown="True" w231 {
              tunnel: [w241 w242] -> w237
              tunnel: w234 -> [w240 w242]
              tunnel: w233 -> [w239 _]
              tunnel: w230 -> [w238 _]
              frame True {
                n98 = invoke class="VI" method="FP.Open"(reference=w239, error in=w240, "State"=w238) -> (error out=w241:errorcluster)  [unwired: 2 in, 4 out]
              }
              frame False {
              }
            }
          }
          frame "Maximize", "Maximized" {
            w243 = T1."Maximized" ("State")
            n99 = property class="VI"(reference=w249, error in=w248) -> (reference out=w246:refnum<vi>, error out=w247:errorcluster, "FP.State"=w245:T1)
            n100 = Not Equal?(x=w245, y=w243) -> (x != y?=w244:bool)
            n101 = case shown="True" w244 {
              tunnel: [w254 w255] -> w250
              tunnel: w247 -> [w253 w255]
              tunnel: w246 -> [w252 _]
              tunnel: w243 -> [w251 _]
              frame True {
                n102 = invoke class="VI" method="FP.Open"(reference=w252, error in=w253, "State"=w251) -> (error out=w254:errorcluster)  [unwired: 2 in, 4 out]
              }
              frame False {
              }
            }
          }
        }
        n103 = call <vilib>:"Add State(s) to Queue__jki_lib_state_machine.vi"("State(s) in (\"\")"=w190) -> ("States Out"=w189:string)  [unwired: 14 in]
      }
      frame "UI: UpdateContext" {
        n104 = Unbundle By Name(w260) -> ("Context[]"=w257:T4)
        n105 = for {
          tunnel: w257 -> [w264] mode=indexing
          tunnel: [w263] -> w256 mode=indexing
          n106 = Unbundle By Name(w264) -> ("Display"=w263:string)
        }
        n107 = property on="Context" class="Ring (strict)"(error in=w259, "Strings []"=w256) -> (error out=w258:errorcluster)  [unwired: 1 in, 1 out]
        n108 = call <vilib>:"Add State(s) to Queue__jki_lib_state_machine.vi"("State(s) in (\"\")"=w262) -> ("States Out"=w261:string)  [unwired: 14 in]
      }
      frame "UI: UpdateSourceFiles" {
        n109 = Unbundle By Name(w281) -> ("SourceFiles[]"=w280:path[])
        n110 = Path To String(path=w280) -> (string=w277:string[])
        n111 = Build Array(w277) -> (w276:string[][])
        n112 = control-ref of="VITree"() -> (w274:refnum<vi>)
        n113 = Transpose 2D Array(2D array=w276) -> (transposed array=w275:string[][])
        n114 = call <userlib>:"MGI Populate Tree with Delimited Strings.vi"("Use Child Only?"=TRUE, "Default Symbol"=14, "error in (no error)"=w279, "Delimiter"="\\", "Items (Delimited)"=w275, "Tree Control"=w274) -> ("error out"=w278:errorcluster, "Tree Control Dup"=w270:refnum<vi>)  [unwired: 3 in, 1 out]
        n115 = property class="Tree"(reference=w270, error in=w278) -> (reference out=w266:refnum<vi>, error out=w268:errorcluster, "All Tags"=w265:string[])
        n116 = for {
          tunnel: [w284] -> w269 mode=indexing
          tunnel: w268 -> [w293]
          tunnel: w266 -> [w292]
          tunnel: w265 -> [w286] mode=indexing
          n117 = property class="Tree"(reference=w292, error in=w293, "Active Item Tag"=w286) -> (reference out=w290:refnum<vi>, error out=w291:errorcluster, "Child-Only?"=w289:bool)
          n118 = Select(t=21, s=w289, f=14) -> (s? t:f=w285:i32)
          n119 = property class="Tree"(reference=w290, error in=w291, "Active Item Tag"=w286, "Glyph"=w285) -> (error out=w284:errorcluster)  [unwired: 1 out]
        }
        n120 = Merge Errors(w269) -> (w267:errorcluster)
        n121 = call <vilib>:"Add State(s) to Queue__jki_lib_state_machine.vi"("State(s) in (\"\")"=w283) -> ("States Out"=w282:string)  [unwired: 14 in]
      }
      frame "UI: UpdateUnCoveredDiagram" {
        n122 = Unbundle By Name(w300) -> ("Uncovered Diagrams"=w296:refnum<vi>[])
        n123 = for {
          tunnel: w298 -> [w308]
          tunnel: [w305] -> w297 mode=indexing
          tunnel: w296 -> [w306] mode=indexing
          tunnel: [w303] -> w295 mode=indexing
          n124 = property class="Diag"(reference=w306, error in=w308) -> (error out=w307:errorcluster, "UID"=w304:i32)  [unwired: 1 out]
          n125 = Format Into String(error in=w307, w304) -> (resulting string=w303:string, error out=w305:errorcluster)  [unwired: 2 in]
        }
        n126 = Merge Errors(w297) -> (w294:errorcluster)
        n127 = property on="UnCoveredDiagram" class="LstBox (strict)"(error in=w294, "Item Names"=w295) -> (error out=w299:errorcluster)  [unwired: 1 in, 1 out]
        n128 = call <vilib>:"Add State(s) to Queue__jki_lib_state_machine.vi"("State(s) in (\"\")"=w302) -> ("States Out"=w301:string)  [unwired: 14 in]
      }
      frame "---------- Macro ----------" {
        # "Do not put any code in this frame.\n(It is a separator no-op. You can make a copy of this frame to create a new Macro frame)"
        n129 = call <vilib>:"Add State(s) to Queue__jki_lib_state_machine.vi"("State(s) in (\"\")"=w312) -> ("States Out"=w311:string)  [unwired: 14 in]
      }
      frame "Macro: Initialize" {
        w313 = "Data: Initialize\nInitialize Core Data\nUI: Initialize\nUI: Front Panel State >> Open\n# NonFrameworkCode\nCC: GetAllContext\nUI: UpdateContext\nUI: UpdateSourceFiles\nCC: GetCodePercentage\nUI: UpdateUnCoveredDiagram"  # Data: Initialize Initialize Core Data UI: Initialize UI: Front Panel State >> Open # NonFrameworkCode CC: GetAllContext UI: UpdateContext UI: UpdateSourceFiles CC: GetCodePercentage UI: UpdateUnCoveredDiagram
        # "Initialization Macro\n(This is called once, when the VI starts)"
        n130 = call <vilib>:"Add State(s) to Queue__jki_lib_state_machine.vi"("State(s) in Front (\"\")"=w313, "State(s) in (\"\")"=w317) -> ("States Out"=w316:string)  [unwired: 13 in]
      }
      frame "Macro: Exit" {
        # "Exit Macro\n(This is called once, when the VI exits)"
        n131 = Unbundle By Name(w324) -> ("Core.Close Panel on Exit?"=w323:bool)
        n132 = Select(t="UI: Front Panel State >> Close", s=w323, f="") -> (s? t:f=w320:string)
        n133 = call <vilib>:"Add State(s) to Queue__jki_lib_state_machine.vi"("State(s) in (\"\")"=w320, "State(s) at Back (\"\")"="Data: Cleanup\nExit") -> ("States Out"=w318:string)  [unwired: 13 in]
        n134 = call <vilib>:"Add State(s) to Queue__jki_lib_state_machine.vi"("State(s) in Front (\"\")"=w318, "State(s) in (\"\")"=w327) -> ("States Out"=w326:string)  [unwired: 13 in]
      }
      frame "---------- CodeCoverage ----------" {
        # "Template Separator\n(You can make a copy of, or modify, this frame)"
        n135 = call <vilib>:"Add State(s) to Queue__jki_lib_state_machine.vi"("State(s) in (\"\")"=w331) -> ("States Out"=w330:string)  [unwired: 14 in]
      }
      frame "CC: GetAllContext" {
        n136 = Unbundle By Name(w343) -> ("Context[]"=w342:T4)
        n137 = call "AllContexts.vi"("error in (no error)"=w344) -> ("Context[]"=w336:string[], "Project[]"=w335:string[], "ProjectPath[]"=w334:path[], "error out"=w339:errorcluster)  [unwired: 11 in]
        n138 = Index Array(array=w342) -> (element=w338:T3)  [unwired: 1 in]
        n139 = call <vilib>:"Clear Errors.vi"("error in (no error)"=w339) -> ("error out"=w340:errorcluster)  [unwired: 5 in, 1 out]
        n140 = for {
          tunnel: w338 -> [w354]
          tunnel: [w353] -> w337 mode=indexing
          tunnel: w336 -> [w350] mode=indexing
          tunnel: w335 -> [w351] mode=indexing
          tunnel: w334 -> [w347] mode=indexing
          n141 = call <vilib>:"Space Constant.vi"() -> ("String"=w349:string)
          n142 = Concatenate Strings(w351, w349, w350) -> (w352:string)
          n143 = call <vilib>:"Trim Whitespace.vi"("string"=w352) -> ("trimmed string"=w348:string)  [unwired: 1 in]
          n144 = Bundle By Name(cluster=w354, "Context"=w350, "Project"=w351, "Display"=w348, "ProjectPath"=w347) -> (w353:T3)
        }
        n145 = Build Array (concatenate)(T3 {"Context"="", "Project"="", "Display"="<Empty>", "ProjectPath"=path ""} ("array"), w337) -> (w333:T4)
        n146 = Bundle By Name(cluster=w343, "Context[]"=w333) -> (w341:T5)
        n147 = call <vilib>:"Add State(s) to Queue__jki_lib_state_machine.vi"("State(s) in (\"\")"=w346) -> ("States Out"=w345:string)  [unwired: 14 in]
      }
      frame "CC: GetCodePercentage" {
        n148 = Unbundle By Name(w356) -> ("ActiveContext"=w355:string)
        n149 = property on="VITree" class="Tree (strict)"(error in=w359) -> (error out=w358:errorcluster, "All Tags"=w357:string[])  [unwired: 1 in, 1 out]
        n150 = for {
          tunnel: [w366] -> w360
          tunnel: w358 -> [w371]
          tunnel: w357 -> [w370] mode=indexing
          tunnel: w355 -> [w363]
          n151 = property on="VITree" class="Tree (strict)"(error in=w371, "Active Item Tag"=w370) -> (error out=w369:errorcluster, "Child-Only?"=w368:bool)  [unwired: 1 in, 1 out]
          n152 = case shown="True" w368 {
            tunnel: [w372 w382] -> w367
            tunnel: w370 -> [_ w381]
            tunnel: w369 -> [w372 w379]
            tunnel: [_ w375] -> w364
            tunnel: w363 -> [_ w374]
            frame False {
            }
            frame True {
              n153 = String To Path(string=w381) -> (path=w380:path)
              n154 = invoke class="App" method="CodeCov.VIPercentage"(error in=w379, "contextName"=w374, "covPercent"=w380) -> (error out=w382:errorcluster, "covPercent"=w377:dbl, "infoFound"=w378:bool)  [unwired: 4 in, 4 out]
              n155 = Number To Fractional String(number=w377) -> (F-format string=w376:string)  [unwired: 3 in]
              n156 = Select(t=w376, s=w378, f="NA") -> (s? t:f=w375:string)
            }
          }
          n157 = property on="VITree" class="Tree (strict)"(error in=w367, "ActiveColNum"=1 ("Active Cell:Active Column Number"), "Cell String"=w364) -> (error out=w366:errorcluster)  [unwired: 1 in, 1 out]
        }
        n158 = call <vilib>:"Add State(s) to Queue__jki_lib_state_machine.vi"("State(s) in (\"\")"=w362) -> ("States Out"=w361:string)  [unwired: 14 in]
      }
      frame "CC: GetUnCoveredDiagram" {
        n159 = Unbundle By Name(w389) -> ("ActiveVI"=w384:string)
        n160 = Empty String/Path?(string/path=w384) -> (empty?=w383:bool)
        n161 = case shown="False" w383 {
          tunnel: w390 -> [w399 w409]
          tunnel: [w396 w409] -> w388
          tunnel: [w395 _] -> w386
          tunnel: [w394 _] -> w385
          tunnel: w384 -> [w393 _]
          frame False {
            n162 = property on="VITree" class="Tree (strict)"(error in=w399, "Active Item Tag"=w393) -> (error out=w398:errorcluster, "Child-Only?"=w397:bool)  [unwired: 1 in, 1 out]
            n163 = case shown="True" w397 {
              tunnel: [w400 w408] -> w396
              tunnel: w393 -> [_ w407]
              tunnel: w398 -> [w400 w406]
              tunnel: w393 -> [_ _]
              tunnel: [_ w402] -> w395
              tunnel: [_ w401] -> w394
              frame False {
              }
              frame True {
                n164 = String To Path(string=w407) -> (path=w404:path)
                n165 = Open VI Reference(vi path=w404, error in (no error)=w406) -> (vi reference=w403:refnum<vi>, error out=w405:errorcluster)  [unwired: 4 in]
                n166 = invoke class="VI" method="CodeCov.UnrunDiags"(reference=w403, error in=w405) -> (reference out=w401:refnum<vi>, error out=w408:errorcluster, "unrunDiags"=w402:refnum<vi>[])  [unwired: 2 in, 1 out]
              }
            }
          }
          frame True {
          }
        }
        n167 = Bundle By Name(cluster=w389, "ActiveVIRef"=w385, "Uncovered Diagrams"=w386) -> (w387:T5)
        n168 = call <vilib>:"Add State(s) to Queue__jki_lib_state_machine.vi"("State(s) in (\"\")"=w392) -> ("States Out"=w391:string)  [unwired: 14 in]
      }
      frame "CC: CleanUnCoveredDiagram" {
        n169 = Unbundle By Name(w419) -> ("ActiveVIRef"=w411:refnum<vi>, "Uncovered Diagrams"=w416:refnum<vi>[])
        n170 = Close Reference(reference=w416, error in (no error)=w417) -> (error out=w413:errorcluster)
        n171 = Close Reference(reference=w411, error in (no error)=w413) -> (error out=w412:errorcluster)
        n172 = call <vilib>:"Clear Errors.vi"("error in (no error)"=w412) -> ("error out"=w410:errorcluster)  [unwired: 5 in, 1 out]
        n173 = Bundle By Name(cluster=w419, "ActiveVIRef"=refnum<vi> refnum, "Uncovered Diagrams"=refnum<vi>[] []) -> (w418:T5)
        n174 = call <vilib>:"Add State(s) to Queue__jki_lib_state_machine.vi"("State(s) in (\"\")"=w421) -> ("States Out"=w420:string)  [unwired: 14 in]
      }
      frame "---------- New Category ----------" {
        # "Template Separator\n(You can make a copy of, or modify, this frame)"
        n175 = call <vilib>:"Add State(s) to Queue__jki_lib_state_machine.vi"("State(s) in (\"\")"=w425) -> ("States Out"=w424:string)  [unwired: 14 in]
      }
      frame "New Category: 1" {
        n176 = call <vilib>:"Add State(s) to Queue__jki_lib_state_machine.vi"("State(s) in (\"\")"=w429) -> ("States Out"=w428:string)  [unwired: 14 in]
      }
      frame "New Category: 2" {
        # "Your code here.\n(You can make a copy of, or modify, this frame)"
        n177 = call <vilib>:"Add State(s) to Queue__jki_lib_state_machine.vi"("State(s) in (\"\")"=w433) -> ("States Out"=w432:string)  [unwired: 14 in]
      }
      frame "Source: GetSourceFiles" {
        n178 = Unbundle By Name(w442) -> ("SourcePath"=w439:path)
        n179 = call <vilib>:"Recursive File List.vi"("pattern"="*.vi", "error in (no error)"=w441, "Folder Path"=w439) -> ("error out"=w440:errorcluster, "All Files in Dir"=w435:path[])  [unwired: 4 in, 3 out]
        n180 = case shown="No Error" w440 {
          selector: w440 -> [w446 _]
          tunnel: [w446 errorcluster {"status"=FALSE, "code"=0, "source"=""} ("error IO")] -> w436
          tunnel: w435 -> [w445 w448]
          tunnel: [w445 w448] -> w434
          frame No Error {
          }
          frame Error {
          }
        }
        n181 = Bundle By Name(cluster=w442, "SourceFiles[]"=w434) -> (w437:T5)
        n182 = call <vilib>:"Add State(s) to Queue__jki_lib_state_machine.vi"("State(s) in (\"\")"=w444) -> ("States Out"=w443:string)  [unwired: 14 in]
      }
      frame "CC: GetMeasuredVIs" {
        n183 = Unbundle By Name(w454) -> ("ActiveContext"=w453:string)
        n184 = invoke class="App" method="CodeCov.AllVIs"(error in=w456, "contextName"=w453) -> (error out=w455:errorcluster, "measuredVIs"=w450:path[])  [unwired: 3 in, 3 out]
        n185 = Path To String(path=w450) -> (string=w452:string[])
        n186 = To Lower Case(string=w452) -> (all lower case string=w451:string[])
        n187 = String To Path(string=w451) -> (path=w449:path[])
        n188 = Bundle By Name(cluster=w454, "SourceFiles[]"=w449) -> (w457:T5)
        n189 = call <vilib>:"Add State(s) to Queue__jki_lib_state_machine.vi"("State(s) in (\"\")"=w459) -> ("States Out"=w458:string)  [unwired: 14 in]
      }
    }
  }
